vi "Point Tool Histogram Filter 2.vi"(4 "Range":cluster{"Lower value":sgl, "Upper value":sgl}={"Lower value"=162.0, "Upper value"=255.0}, 6 "Color threshold limits":T1, 7 "Filter Selection":string(combo)="Pattern_matching", 8 "error in":errorcluster, 9 "RGB":T2, 10 "Subtraction Image":path, 11 "Main_Gray":T2) -> (0 "error out":errorcluster, 1 "Main_Gray Out":T2)   [LabVIEW 2017]
uses:
  <vilib>/vision/Image Controls.llb/IMAQ Image.ctl
  <vilib>/vision/NI_Vision_Development_Module.lvlib
panel:
  out "Image":T2(plugin-control)
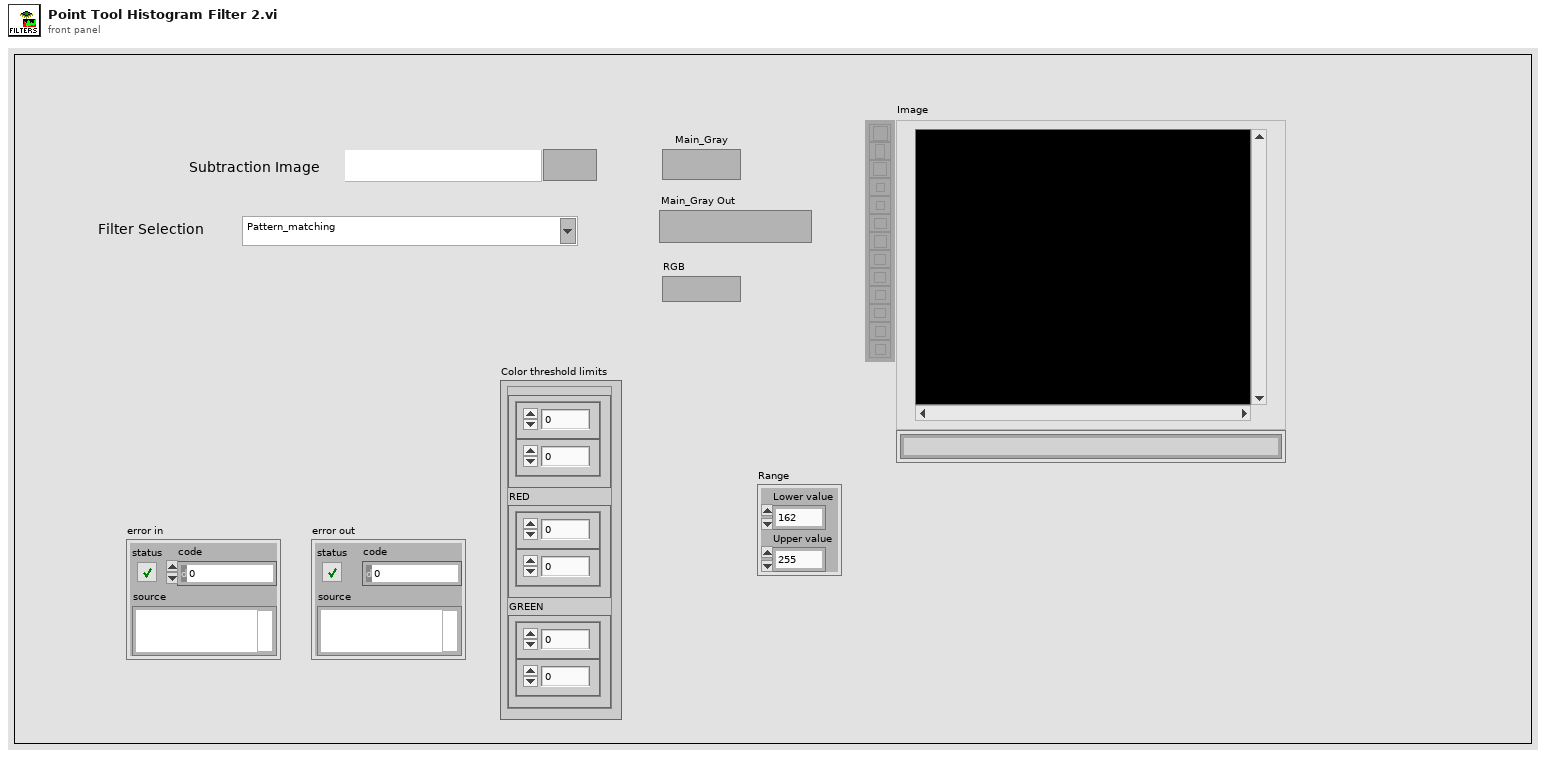
[diagram p1: front panel]
types:
  T1 = cluster{"BLUE":cluster{"Numeric Control":dbl, "Numeric Control":dbl}, "RED":cluster{"Numeric Control":dbl, "Numeric Control":dbl}, "GREEN":cluster{"Numeric Control":dbl, "Numeric Control":dbl}}
  T2 = typedef "IMAQ Image.ctl" = refnum<image>
  T3 = enum32{"Linear", "Log", "Exp", "Square", "Square root", "Power X", "Power 1/X"}
  T4 = typedef "Image Type" = u32
  T5 = cluster{"histogram":u32[], "Minimal Value":sgl, "Maximal Value":sgl, "Starting Value":sgl, "Interval Width":sgl, "Mean Value":sgl, "Standard  Variation":sgl, "Area (pixels)":i32}
  T6 = cluster{"Numeric Control":dbl, "Numeric Control":dbl}
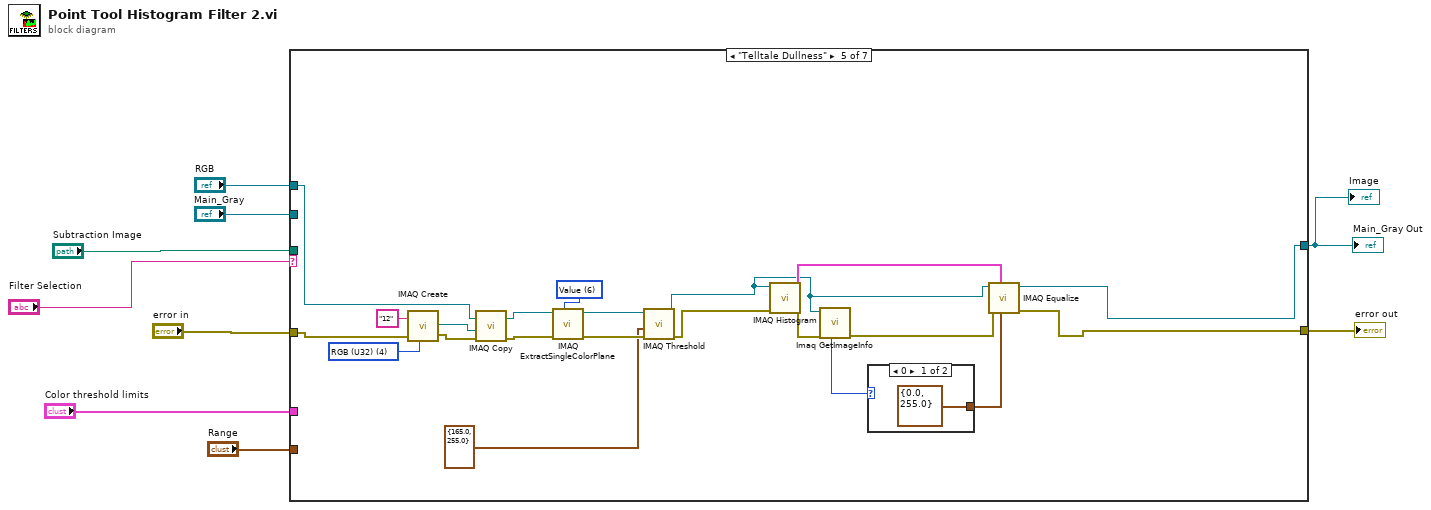
[diagram p0: block diagram]
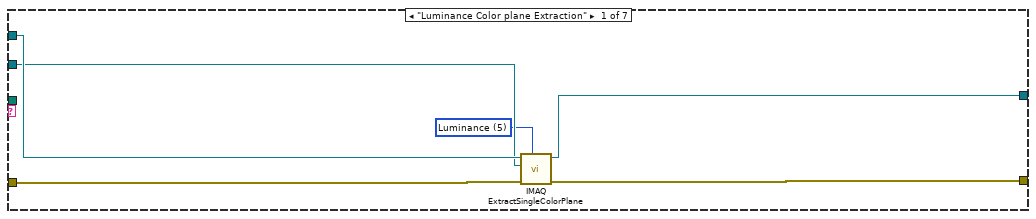
[diagram p2: hidden frame]
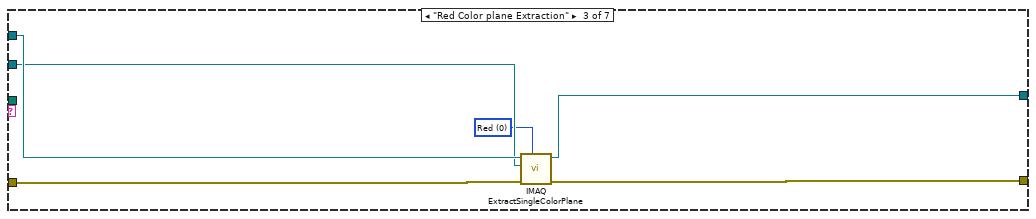
[diagram p4: hidden frame]
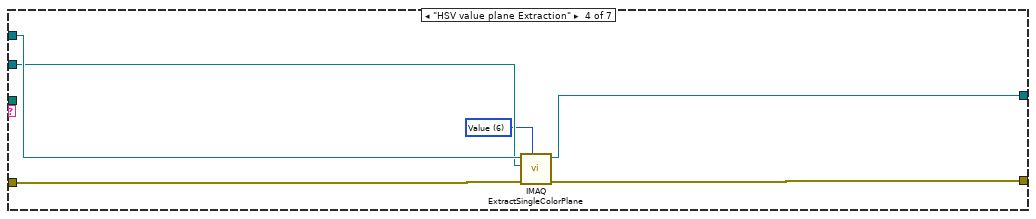
[diagram p5: hidden frame]
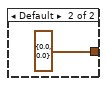
[diagram p6: hidden frame]
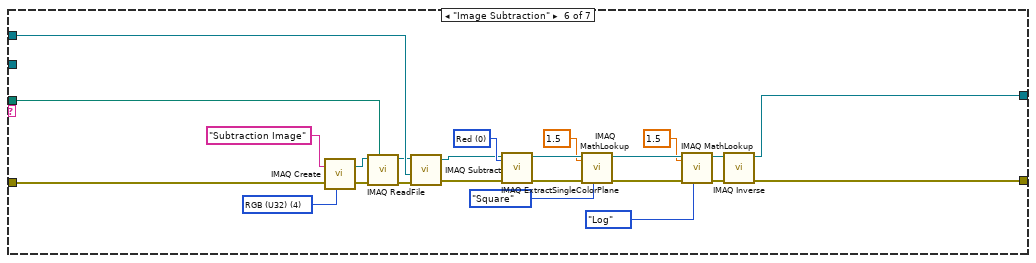
[diagram p7: hidden frame]
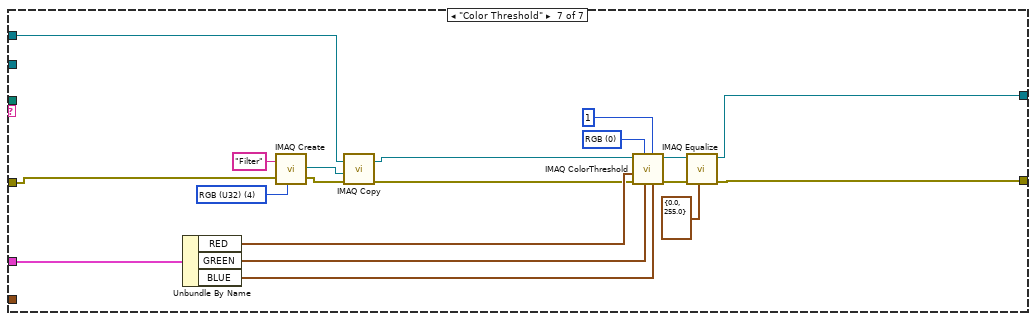
[diagram p8: hidden frame]
diagram:
  n1 = case shown="\"Telltale Dullness\"" "Filter Selection" {
    tunnel: [w14 w17 w22 w28 w40 w76 w90] -> w9
    tunnel: "RGB" -> [w13 w16 w21 w27 w32 w75 w78]
    tunnel: "Subtraction Image" -> [_ _ _ _ _ w74 _]
    tunnel: [w12 w16 w20 w26 w39 w73 w85] -> w7
    tunnel: "error in" -> [w15 w17 w23 w29 w34 w53 w83]
    tunnel: "Main_Gray" -> [w11 _ w19 w25 _ _ _]
    tunnel: "Color threshold limits" -> [_ _ _ _ _ _ w89]
    tunnel: "Range" -> [_ _ _ _ _ _ _]
    frame "Luminance Color plane Extraction" {
      w10 = 5 items=["Red", "Green", "Blue", "Hue", "Saturation", "Luminance", "Value", "Intensity"] ("Color Plane")
      n2 = call "IMAQ ExtractSingleColorPlane"("Color Plane"=w10, "error in (no error)"=w15, "Image Dst"=w11, "Image Src"=w13) -> ("error out"=w14:errorcluster, "Image Dst Out"=w12:T2)  [unwired: 6 in]
    }
    frame "False", Default {
    }
    frame "Red Color plane Extraction" {
      w18 = 0 items=["Red", "Green", "Blue", "Hue", "Saturation", "Luminance", "Value", "Intensity"] ("Color Plane")
      n3 = call "IMAQ ExtractSingleColorPlane"("Color Plane"=w18, "error in (no error)"=w23, "Image Dst"=w19, "Image Src"=w21) -> ("error out"=w22:errorcluster, "Image Dst Out"=w20:T2)  [unwired: 6 in]
    }
    frame "HSV value plane Extraction" {
      w24 = 6 items=["Red", "Green", "Blue", "Hue", "Saturation", "Luminance", "Value", "Intensity"] ("Color Plane")
      n4 = call "IMAQ ExtractSingleColorPlane"("Color Plane"=w24, "error in (no error)"=w29, "Image Dst"=w25, "Image Src"=w27) -> ("error out"=w28:errorcluster, "Image Dst Out"=w26:T2)  [unwired: 6 in]
    }
    frame "Telltale Dullness" {
      w36 = T4 4 items=["Grayscale (U8)", "Grayscale (I16)", "Grayscale (SGL)", "Complex (CSG)", "RGB (U32)", "HSL (U32)", "RGB (U64)", "Grayscale (U16)"] ("Image Type")
      w50 = 6 items=["Red", "Green", "Blue", "Hue", "Saturation", "Luminance", "Value", "Intensity"] ("Color Plane")
      n5 = call "IMAQ Create"("Image Name"="12", "Image Type"=w36, "error in (no error)"=w34) -> ("New Image"=w35:T2, "error out"=w38:errorcluster)  [unwired: 2 in]
      n6 = call "IMAQ Copy"("error in (no error)"=w38, "Image Dst"=w35, "Image Src"=w32) -> ("error out"=w33:errorcluster, "Image Dst Out"=w31:T2)  [unwired: 3 in]
      n7 = call "IMAQ ExtractSingleColorPlane"("Color Plane"=w50, "error in (no error)"=w33, "Image Src"=w31) -> ("error out"=w49:errorcluster, "Image Dst Out"=w48:T2)  [unwired: 1 in, 6 out]
      n8 = call "IMAQ Threshold"("error in (no error)"=w49, "Range"=cluster{"Lower value":sgl, "Upper value":sgl} {"Lower value"=165.0, "Upper value"=255.0}, "Image Src"=w48) -> ("error out"=w42:errorcluster, "Image Dst Out"=w41:T2)  [unwired: 3 in, 4 out]
      n9 = call "IMAQ Histogram"("error in (no error)"=w42, "Image"=w41) -> ("error out"=w45:errorcluster, "Histogram Report"=w47:T5)  [unwired: 3 in, 5 out]
      n10 = call "Imaq GetImageInfo"("error in (no error)"=w45, "Image"=w41) -> ("error out"=w44:errorcluster, "Image Type"=w46:T4)  [unwired: 8 out]
      n11 = case shown="0" w46 {
        tunnel: [cluster{"Minimum":sgl, "Maximum":sgl} {"Minimum"=0.0, "Maximum"=255.0} ("Range") cluster{"Minimum":sgl, "Maximum":sgl} {"Minimum"=0.0, "Maximum"=0.0} ("Range")] -> w43
        frame 0 {
        }
        frame Default {
        }
      }
      n12 = call "IMAQ Equalize"("Range"=w43, "Histogram Report"=w47, "error in (no error)"=w44, "Image Src"=w41) -> ("error out"=w40:errorcluster, "Image Dst Out"=w39:T2)  [unwired: 2 in, 4 out]
    }
    frame "Image Subtraction" {
      w60 = 0 items=["Red", "Green", "Blue", "Hue", "Saturation", "Luminance", "Value", "Intensity"] ("Color Plane")
      w69 = T4 4 items=["Grayscale (U8)", "Grayscale (I16)", "Grayscale (SGL)", "Complex (CSG)", "RGB (U32)", "HSL (U32)", "RGB (U64)", "Grayscale (U16)"] ("Image Type")
      n13 = call "IMAQ Create"("Image Name"="Subtraction Image", "Image Type"=w69, "error in (no error)"=w53) -> ("New Image"=w71:T2, "error out"=w72:errorcluster)  [unwired: 2 in]
      n14 = call "IMAQ ReadFile"("File Path"=w74, "error in (no error)"=w72, "Image"=w71) -> ("error out"=w68:errorcluster, "Image Out"=w67:T2)  [unwired: 4 in, 3 out]
      n15 = call "IMAQ Subtract"("Image Src A"=w67, "Image Src B"=w75, "error in (no error)"=w68) -> ("Image Dst Out"=w55:T2, "error out"=w54:errorcluster)  [unwired: 4 in]
      n16 = call "IMAQ ExtractSingleColorPlane"("Color Plane"=w60, "error in (no error)"=w54, "Image Src"=w55) -> ("error out"=w61:errorcluster, "Image Dst Out"=w62:T2)  [unwired: 1 in, 6 out]
      n17 = call "IMAQ MathLookup"("Operator"=T3."Square", "X Value"=sgl 1.5, "error in (no error)"=w61, "Image Src"=w62) -> ("error out"=w63:errorcluster, "Image Dst Out"=w64:T2)  [unwired: 3 in, 3 out]
      n18 = call "IMAQ MathLookup"("Operator"=T3."Log", "X Value"=sgl 1.5, "error in (no error)"=w63, "Image Src"=w64) -> ("error out"=w65:errorcluster, "Image Dst Out"=w66:T2)  [unwired: 3 in, 3 out]
      n19 = call "IMAQ Inverse"("error in (no error)"=w65, "Image Src"=w66) -> ("error out"=w76:errorcluster, "Image Dst Out"=w73:T2)  [unwired: 2 in, 6 out]
    }
    frame "Color Threshold" {
      w80 = T4 4 items=["Grayscale (U8)", "Grayscale (I16)", "Grayscale (SGL)", "Complex (CSG)", "RGB (U32)", "HSL (U32)", "RGB (U64)", "Grayscale (U16)"] ("Image Type")
      w95 = u16 0 items=["RGB", "HSL", "HSV", "HSI"] ("Color Mode (Color Threshold 1)")
      n20 = Unbundle By Name(w89) -> ("RED"=w88:T6, "GREEN"=w87:T6, "BLUE"=w86:T6)
      n21 = call "IMAQ Create"("Image Name"="Filter", "Image Type"=w80, "error in (no error)"=w83) -> ("New Image"=w79:T2, "error out"=w84:errorcluster)  [unwired: 2 in]
      n22 = call "IMAQ Copy"("error in (no error)"=w84, "Image Dst"=w79, "Image Src"=w78) -> ("error out"=w82:errorcluster, "Image Dst Out"=w77:T2)  [unwired: 3 in]
      n23 = call "IMAQ ColorThreshold"("Blue or Luma or Val or Inten Range"=w86, "Replace Value"=1, "Green or Sat Range"=w87, "Color Mode"=w95, "error in (no error)"=w82, "Red or Hue Range"=w88, "Image Src"=w77) -> ("error out"=w91:errorcluster, "Image Dst Out"=w92:T2)  [unwired: 1 in, 2 out]
      n24 = call "IMAQ Equalize"("Range"=cluster{"Minimum":sgl, "Maximum":sgl} {"Minimum"=0.0, "Maximum"=255.0}, "error in (no error)"=w91, "Image Src"=w92) -> ("error out"=w90:errorcluster, "Image Dst Out"=w85:T2)  [unwired: 3 in, 4 out]
    }
  }
  "Main_Gray Out" <- w7
  "error out" <- w9
  "Image" <- w7
